vi "Draw Joystick Axes.vi"(9 "Size":cluster{"X":u32, "Y":u32}, 11 "Mouse":T1) -> (1 "JS Coords":cluster{"X":dbl, "Y":dbl}, 3 "Arcade Inputs":picture)   [LabVIEW 2020]
uses:
  <vilib>/Utility/miscctls.llb/LVMouseTypeDef.ctl
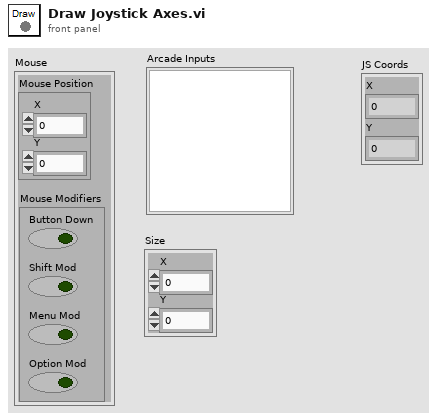
[diagram p1: front panel]
types:
  T1 = typedef "LVMouseTypeDef.ctl" = cluster{"Mouse Position":cluster{"X":i32, "Y":i32}, "Mouse Modifiers":cluster{"Button Down":bool, "Shift Mod":bool, "Menu Mod":bool, "Option Mod":bool}}
  T2 = cluster{"Button Down":bool, "Shift Mod":bool, "Menu Mod":bool, "Option Mod":bool}
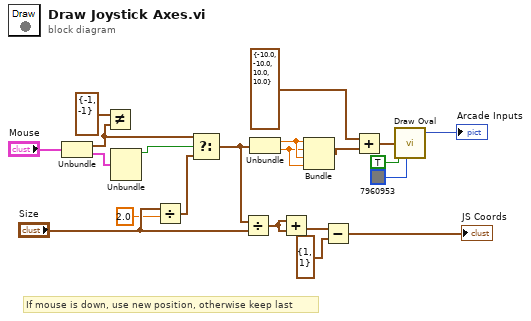
[diagram p0: block diagram]
diagram:
  # "If mouse is down, use new position, otherwise keep last"
  n1 = Unbundle("Mouse") -> ("Mouse Position"=w7:cluster{"X":i32, "Y":i32}, "Mouse Modifiers"=w6:T2)
  n2 = Not Equal?(x=cluster{"X":i32, "Y":i32} {"X"=-1, "Y"=-1}, y=w7) -> ()  [unwired: 1 out]
  n3 = Unbundle(w6) -> ("Button Down"=w5:bool)  [unwired: 3 out]
  n4 = Divide(x="Size", y=2.0) -> (x/y=w1:cluster{"X":dbl, "Y":dbl})
  n5 = Select(t=w7, s=w5, f=w1) -> (s? t:f=w4:cluster{"X":dbl, "Y":dbl})
  n6 = Divide(x=w4, y="Size") -> (x/y=w11:cluster{"X":dbl, "Y":dbl})
  n7 = Unbundle(w4) -> ("X"=w18:dbl, "Y"=w17:dbl)
  n8 = Add(x=w11, y=w11) -> (x+y=w10:cluster{"X":dbl, "Y":dbl})
  n9 = Bundle("X"=w18, "Y"=w17, "X"=w18, "Y"=w17) -> (w16:cluster{"X":dbl, "Y":dbl, "X":dbl, "Y":dbl})  [unwired: 1 in]
  n10 = Subtract(x=w10, y=cluster{"X":i32, "Y":i32} {"X"=1, "Y"=1} ("x")) -> (x-y=→"JS Coords":cluster{"X":dbl, "Y":dbl})
  n11 = Add(x=cluster{"X":dbl, "Y":dbl, "X":dbl, "Y":dbl} {"X"=-10.0, "Y"=-10.0, "X"=10.0, "Y"=10.0}, y=w16) -> (x+y=w14:cluster{"X":dbl, "Y":dbl, "X":dbl, "Y":dbl})
  n12 = call <vilib>:"Draw Oval.vi"("rect"=w14, "fill?(F)"=TRUE, "color(black)"=u32 7960953) -> ("new picture"=→"Arcade Inputs":picture)  [unwired: 6 in]
